vi "Read Data.vi"(8 "error in (no error)":errorcluster, 11 "KeithleyMeter in":refnum<class "KeithleyMeter.lvclass">) -> (0 "error out":errorcluster, 2 "Data":waveform(dbl)[](array[waveform]), 3 "KeithleyMeter out":refnum<class "KeithleyMeter.lvclass">)   [LabVIEW 2015, in "KeithleyMeter.lvclass"]
uses:
  KeithleyMeter.lvclass
  Instrument/Instrument.lvclass
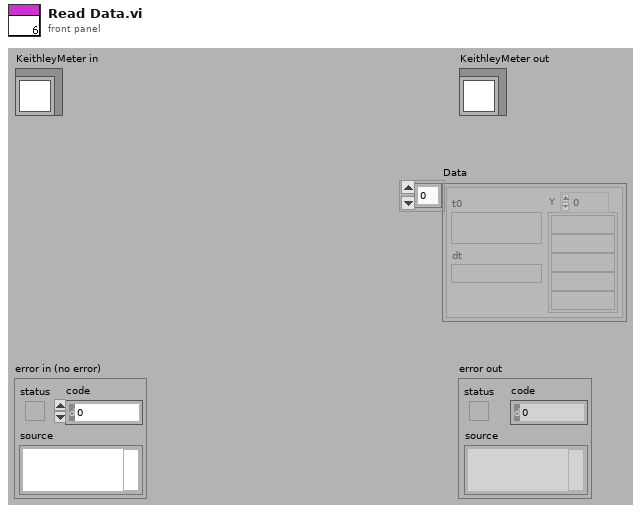
[diagram p1: front panel]
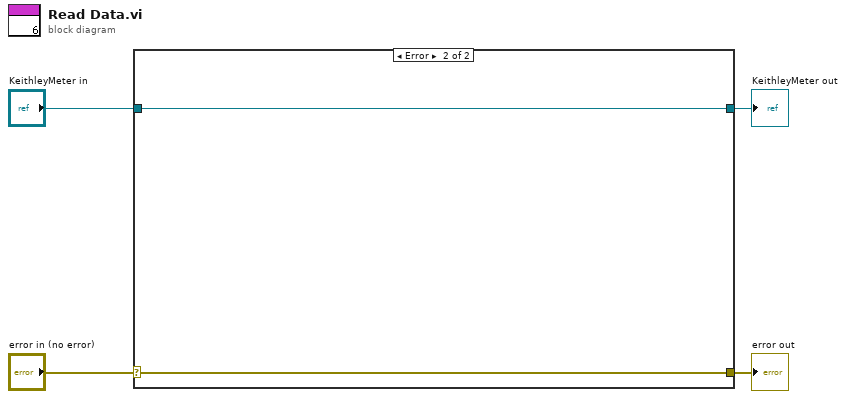
[diagram p0: block diagram]
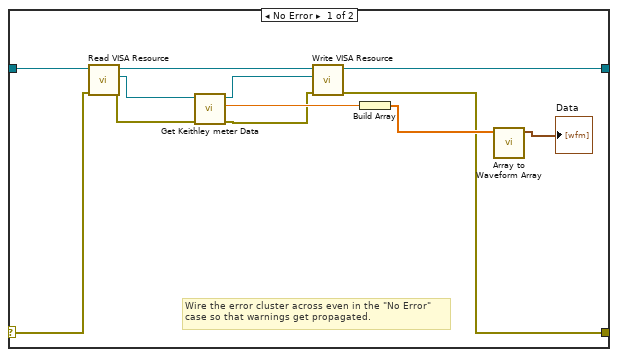
[diagram p2: hidden frame]
diagram:
  n1 = case shown="Error" "error in (no error)" {
    selector: "error in (no error)" -> [w11 w18]
    tunnel: [w6 w18] -> w3
    tunnel: [w14 w17] -> w1
    tunnel: "KeithleyMeter in" -> [w16 w17]
    frame No Error {
      # "Wire the error cluster across even in the \"No Error\"\ncase so that warnings get propagated."
      n2 = call "Read VISA Resource.vi"("error in (no error)"=w11, "Instrument.lvclass in"=w16) -> ("error out"=w10:errorcluster, "VISA Resource"=w13:refnum<visa-resource-name>, "Instrument.lvclass out"=w15:refnum<class "KeithleyMeter.lvclass">)  [unwired: 7 out]
      n3 = call "Get Keithley meter Data.vi"("error in (no error)"=w10, "VISA Resource Name"=w13) -> ("error out"=w7:errorcluster, "Data"=w9:dbl, "VISA Resource Name Out"=w12:refnum<visa-resource-name>)  [unwired: 2 in, 5 out]
      n4 = call "Write VISA Resource.vi"("error in (no error)"=w7, "VISA Resource"=w12, "Instrument.lvclass in"=w15) -> ("error out"=w6:errorcluster, "Instrument.lvclass out"=w14:refnum<class "KeithleyMeter.lvclass">)  [unwired: 7 out]
      n5 = Build Array(w9) -> (w8:dbl[])
      n6 = call "Array to Waveform Array.vi"("Array"=w8) -> ("Waveform"=→"Data":waveform(dbl)[])  [unwired: 10 in]
    }
    frame Error {
    }
  }
  "error out" <- w3
  "KeithleyMeter out" <- w1
